vi "get_ID.vi"(8 "error in (no error)":errorcluster, 11 "Pfeiffer MultiGauge TPG256 in":refnum<class "Pfeiffer MultiGauge TPG256.lvclass">) -> (0 "error out":errorcluster, 2 "ID from Instrument":string, 3 "Pfeiffer MultiGauge TPG256 out":refnum<class "Pfeiffer MultiGauge TPG256.lvclass">)   [LabVIEW 2017, in "Pfeiffer MultiGauge TPG256.lvclass"]
doc: "the vi reads the ID from the instrument"
uses:
  Pfeiffer MultiGauge TPG256.lvclass
  instrument.lvclass
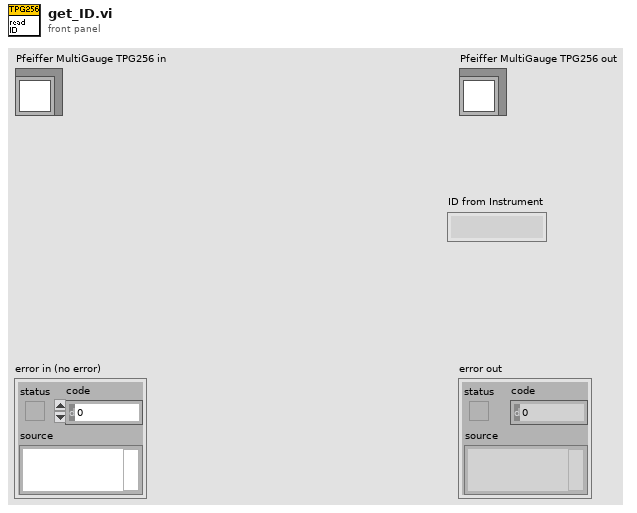
[diagram p1: front panel]
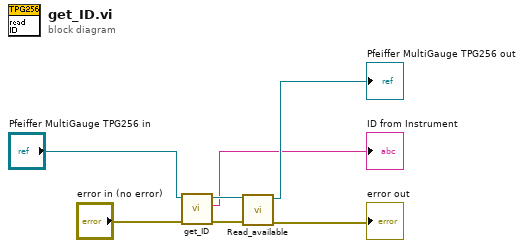
[diagram p0: block diagram]
diagram:
  n1 = call-parent "get_ID.vi"("error in (no error)"="error in (no error)", "instrument in"="Pfeiffer MultiGauge TPG256 in") -> ("error out"=w4:errorcluster, "ID from Instrument"=→"ID from Instrument":string, "instrument out"=w5:refnum<class "Pfeiffer MultiGauge TPG256.lvclass">)  [unwired: 7 in]
  n2 = call-dynamic "Read_available.vi"("error in (no error)"=w4, "instrument in"=w5) -> ("error out"=→"error out":errorcluster, "instrument out"=→"Pfeiffer MultiGauge TPG256 out":refnum<class "Pfeiffer MultiGauge TPG256.lvclass">)  [unwired: 7 in, 1 out]
